vi "Get All Instrument Value(SubVI).vi"(11 "队列输入":refnum<queue>) -> (2 "数组":dbl[](array[numeric]))   [LabVIEW 2019, in "SubVI.lvlib"]
uses:
  SubVI.lvlib
  config.ctl
  Instrument.ctl
  lib/QDInstrument.dll
panel:
  # "(真是通道1，假是通道2)"
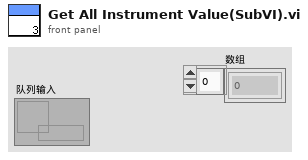
[diagram p1: front panel]
types:
  T1 = typedef "config.ctl" = cluster{"initialize":string, "6221":cluster{"6221 Resource":refnum<visa-resource-name>, "Delta status":bool}, "7001":cluster{"Ch":bool}, "SR830+6221":cluster{"source":u16, "阻抗":dbl, "量程入 4":i32, "量程入 3":i32, "量程入 2":i32, "量程入 1":i32, "电流":dbl, "SR830 2":bool, "SR830 3":bool, "SR830 4":bool, "SR830 1":bool, "VISA 1":refnum<visa-resource-name>, "VISA 2":refnum<visa-resource-name>, "VISA 3":refnum<visa-resource-name>, "VISA 4":refnum<visa-resource-name>, "量程":enum16{"量程每次测量会判定", "量程不变为设定值"}}, "2400":cluster{"2400":bool, "VISA":refnum<visa-resource-name>}, "ch":cluster{"ch str":string, "ch1":bool, "ch2":bool, "布尔":bool}, "error":bool, "数据文件路径":path, "log":cluster{"log路径":path, "log interval":dbl}, "Instrument":T2}
  T2 = typedef "Instrument.ctl" = cluster{"335 Resource":refnum<visa-resource-name>, "Input (0:A)":u16, "Instrument Type":i32, "quantum design":refnum<k24>, "Heater Output (1:1)":u16}
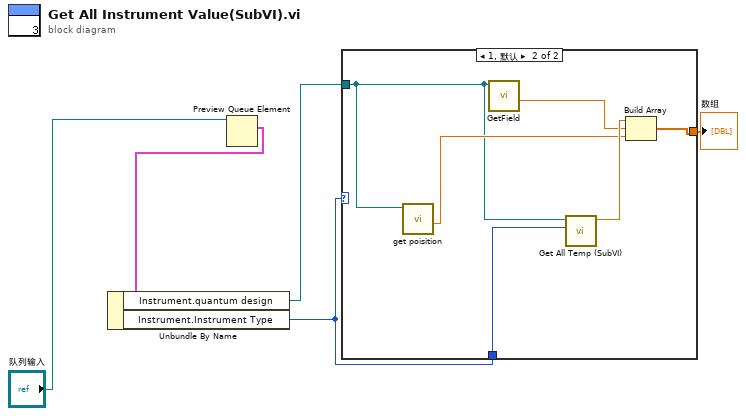
[diagram p0: block diagram]
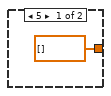
[diagram p2: hidden frame]
diagram:
  n1 = Preview Queue Element(queue="队列输入") -> (element=w3:T1)  [unwired: 2 in, 3 out]
  n2 = Unbundle By Name(w3) -> ("Instrument.quantum design"=w2:refnum<k24>, "Instrument.Instrument Type"=w1:i32)
  n3 = case shown="1, 默认" w1 {
    tunnel: w1 -> [_ w12]
    tunnel: [dbl[] [] w8] -> w5
    tunnel: w2 -> [_ w7]
    frame 5 {
    }
    frame 1, Default {
      n4 = call "get poisition.vi"("Instrument Ref In"=w7) -> ("Position"=w9:dbl)  [unwired: 4 in, 2 out]
      n5 = call "GetField.vi"("Instrument Ref In"=w7) -> ("Field"=w10:dbl)  [unwired: 4 in, 4 out]
      n6 = call "Get All Temp (SubVI).vi"("Instrument Type"=w12, ".NET引用句柄输入"=w7) -> ("Temperature"=w11:dbl)  [unwired: 9 in]
      n7 = Build Array(w11, w10, w9) -> (w8:dbl[])
    }
  }
  "数组" <- w5
